vi "DataLogger_GetParentFolder.vi"(8 "error in (no error)":errorcluster, 11 "Data Logger in":refnum<class "Data Logger.lvclass">) -> (0 "error out":errorcluster, 2 "Parent Folder":path, 3 "Data Logger out":refnum<class "Data Logger.lvclass">)   [LabVIEW 2015, in "Data Logger.lvclass"]
uses:
  Data Logger.lvclass
  Data Logger.lvclass/Data Logger.ctl
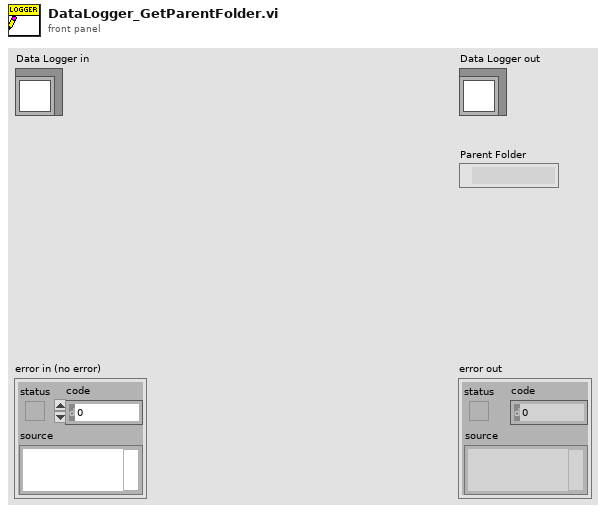
[diagram p1: front panel]
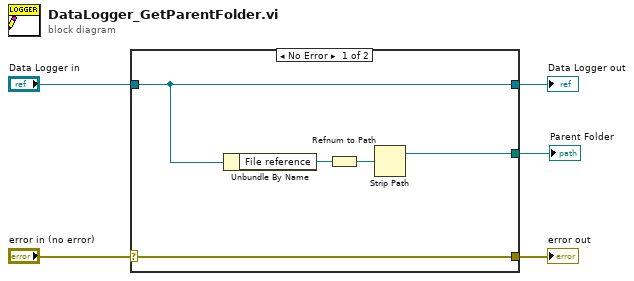
[diagram p0: block diagram]
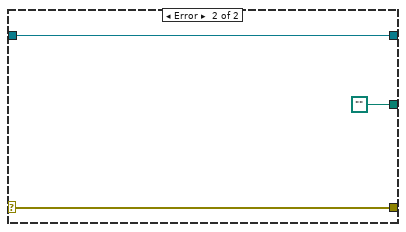
[diagram p2: hidden frame]
diagram:
  n1 = case shown="No Error" "error in (no error)" {
    selector: "error in (no error)" -> [w10 w12]
    tunnel: [w10 w12] -> w4
    tunnel: [w9 w13] -> w2
    tunnel: "Data Logger in" -> [w9 w13]
    tunnel: [w6 path ""] -> w1
    frame No Error {
      n2 = Unbundle By Name(w9) -> ("File reference"=w8:refnum<file>)
      n3 = Refnum to Path(1:w8) -> (0:w7:path)
      n4 = Strip Path(path=w7) -> (stripped path=w6:path)  [unwired: 1 out]
    }
    frame Error {
    }
  }
  "error out" <- w4
  "Data Logger out" <- w2
  "Parent Folder" <- w1
